vi "ModbusCRCTest.vi"() -> ()   [LabVIEW 2018]
uses:
  Common_FPGA_Modbus/FPGAModbus.lvlib
panel:
  out "UInt16":u16 format="%04x"
  in  "CRC":bool
  out "CRC-16/Modbus (HEX)":u8[](array[numeric]) format="%02x"
  in  "Message (HEX)":u8[](array[numeric]) format="%02x"
  # "Calculate CRC-16/Modbus. You can verify results there:\nhttps://crccalc.com/\nDon't forgot to switch input type to HEX"
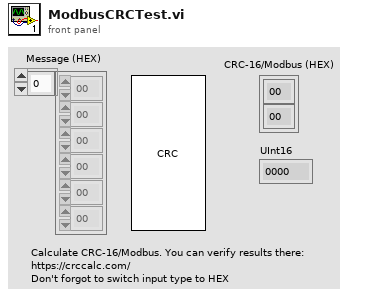
[diagram p1: front panel]
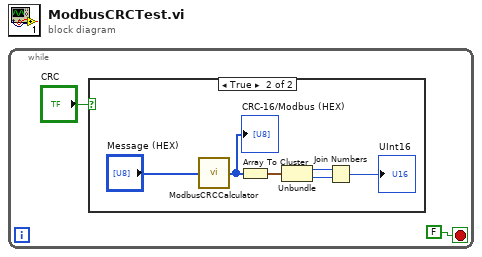
[diagram p0: block diagram]
diagram:
  n1 = while {
    stop <- FALSE stop-if-true
    n2 = case shown="True" "CRC" {
      frame False {
      }
      frame True {
        n3 = call "ModbusCRCCalculator.vi"("Input"="Message (HEX)") -> ("Output"=w7:u8[])
        "CRC-16/Modbus (HEX)" <- w7
        n4 = Array To Cluster(array=w7) -> (cluster=w6:cluster{"Output[0]":u8, "Output[1]":u8})
        n5 = Unbundle(w6) -> ("Output[0]"=w5:u8, "Output[1]"=w3:u8)
        n6 = Join Numbers(hi=w5, lo=w3) -> ((hi.lo)=→"UInt16":u16)
      }
    }
  }
